vi "Parse Data.vi"(8 "error in (no error)":errorcluster, 10 "Received UDP Data":string="$.Data") -> (0 "error out":errorcluster, 2 "Data":string, 3 "Command":string)   [LabVIEW 2021, in "UDP Comms.lvlib"]
uses:
  UDP Comms.lvlib
  dc26f767-2055-49cb-89eb-4c7a1b643544.vi
  <vilib>/JDP Science/JSONtext/Next JSON Value.vi
  <vilib>/JDP Science/JSONtext/String Subset.vi
  <vilib>/JDP Science/JSONtext/Parsing/Advance past next JSON Value (inlined COPY).vi
  <vilib>/JDP Science/JSONtext/Parsing/Advance past whitespace.vi
  <vilib>/JDP Science/JSONtext/Parsing/Advance past String.vi
  <vilib>/JDP Science/JSONtext/Parsing/Advance past Number.vi
  <vilib>/JDP Science/JSONtext/Parsing/Advance past Line Ending.vi
  <vilib>/JDP Science/JSONtext/Parsing/Parse Full Path or Item Name.vi
  <vilib>/JDP Science/JSONtext/Parsing/Advance past Array.vi
  <vilib>/JDP Science/JSONtext/Parsing/Advance past Object.vi
  <vilib>/JDP Science/JSONtext/support/Error Cluster From Code.vi
  <vilib>/JDP Science/JSONtext/Offset/Find Item Locations by Path.vi
  <vilib>/JDP Science/JSONtext/JSON text to Variant.vi
  <vilib>/JDP Science/JSONtext/LVClass Serializer/JSONtext LVClass Serializer.lvclass
  <vilib>/JDP Science/JSONtext/JSONtext.lvlib
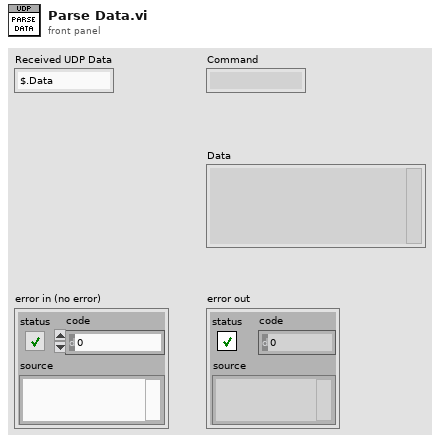
[diagram p1: front panel]
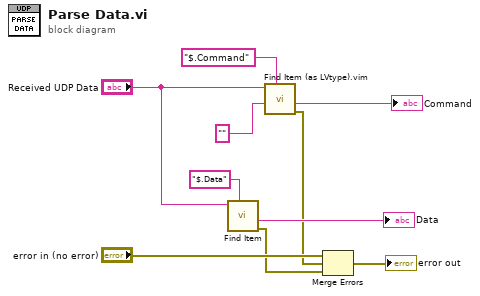
[diagram p0: block diagram]
diagram:
  n1 = call <vilib>:"Find Item.vi"("$Path or Item Name"="$.Data", "JSON"="Received UDP Data") -> ("error out"=w1:errorcluster, "<JSON>"=→"Data":string)  [unwired: 6 in, 2 out]
  n2 = call "Find Item (as LVtype).vim"("$Path or Item Name"="$.Command", "Data Type and Default Value"="" ("$Path or Item Name"), "JSON"="Received UDP Data") -> ("error out"=w2:errorcluster, "Data"=→"Command":string)  [unwired: 5 in, 2 out]
  n3 = Merge Errors("error in (no error)", w2, w1) -> (→"error out":errorcluster)
